vi "Get Default Word.vi"(8 "error in":errorcluster, 11 "label ref":T1 format="%.0x") -> (0 "error out":errorcluster, 2 "default word":u32 format="%032b", 3 "label ref out":T1 format="%.0x")   [LabVIEW 2020, in "AIM ARINC 429 Scripting.lvlib"]
uses:
  AIM ARINC 429 Scripting.lvlib
  <vilib>/NI VeriStand/Custom Device API/Custom Device Item Ref.ctl
  Constants.vi
  <vilib>/NI VeriStand/Custom Device API/Get Item Property (U32).vi
  <vilib>/NI VeriStand/Custom Device API/Custom Device API.lvlib
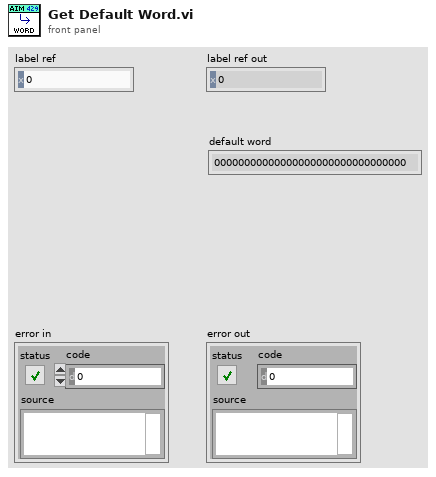
[diagram p1: front panel]
types:
  T1 = typedef "Custom Device API.lvlib/Custom Device Item Ref.ctl" = u64
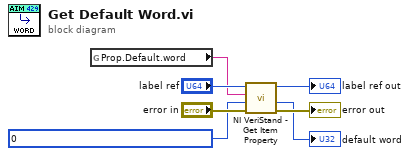
[diagram p0: block diagram]
diagram:
  n1 = global read "Constants.vi" "Prop.Default.word"() -> (w3:string)
  n2 = call-poly <vilib>:"NI VeriStand - Get Item Property.vi"("error in (no error)"="error in", "Default Value"=u32 0, "Property Name"=w3, "Item Ref in"="label ref") -> ("error out"=→"error out":errorcluster, "Value"=→"default word":u32, "Item Ref out"=→"label ref out":T1)  [unwired: 4 in, 1 out]
